vi "Identify.vi"(8 "error in (no error)":errorcluster, 11 "Servo to Compression in":refnum<class "Servo to Compression.lvclass">) -> (0 "error out":errorcluster, 2 "Plugin is Valid":bool, 3 "Servo to Compression out":refnum<class "Servo to Compression.lvclass">)   [LabVIEW 2018, in "Servo to Compression.lvlib" / "Servo to Compression.lvclass"]
uses:
  Servo to Compression.lvclass
  C:/Sequence Automation/Plugins/Measurement Interface.lvlibp/Measurement Interface.lvclass
  C:/Sequence Automation/Plugins/Measurements/Servo MSMT.lvlibp/Servo MSMT.lvclass
  Plugins/Measurement Interface.lvlibp/Private Methods/Measurement Parameters/Read Measurement Parameters.vi
  Plugins/String Database.lvlibp/String Database.lvclass
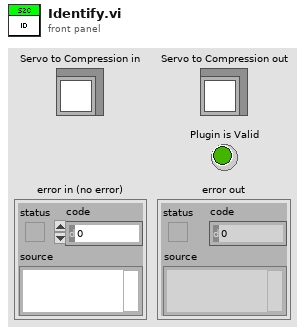
[diagram p1: front panel]
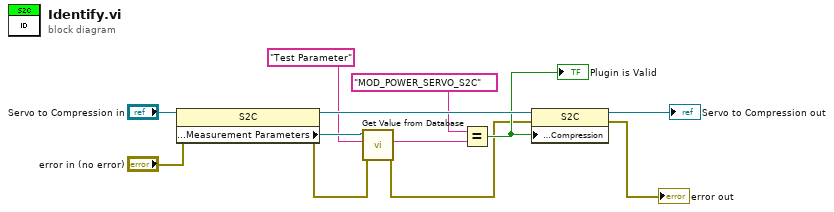
[diagram p0: block diagram]
diagram:
  n1 = property class="S2C"(reference="Servo to Compression in", error in="error in (no error)") -> (reference out=w10:refnum<class "Servo to Compression.lvclass">, error out=w7:errorcluster, "Protected Methods:Measurement Parameters"=w9:refnum<class "String Database.lvclass">)
  n2 = call "Get Value from Database.vi"("error in (no error)"=w7, "Entry Name"="Test Parameter", "Message in"=w9) -> ("error out"=w2:errorcluster, "Entry Value"=w6:string)  [unwired: 5 in, 2 out]
  n3 = Equal?(x="MOD_POWER_SERVO_S2C", y=w6) -> (x = y?=w3:bool)
  "Plugin is Valid" <- w3
  n4 = property class="S2C"(reference=w10, error in=w2, "Protected Methods:Compression"=w3) -> (reference out=→"Servo to Compression out":refnum<class "Servo to Compression.lvclass">, error out=→"error out":errorcluster)
